vi "uc480_SubVI_Example_GetImageSize.vi"(8 "Error In":errorcluster, 11 ".NET (Reference)":refnum<k24>) -> (0 "Error Out":errorcluster, 1 "Height":i32, 2 "Width":i32, 3 ".NET (Reference)":refnum<k24>)   [LabVIEW 2011]
uses:
  C:/Program Files/Thorlabs/Scientific Imaging/DCx Camera Support/Develop/DotNet/uc480DotNet.dll
  Develop/DotNet/uc480DotNet.dll
panel:
  out "SubSampFacVert":i32
  out "Subsampled Width":i32
  out "Binned Width":i32
  out "Subsampled Height":i32
  out "SubSampFacHor":i32
  out "Factored Width":i32
  out "Factored Height":i32
  out "Binned Height":i32
  out "Scaler":dbl
  out "BinFacVert":i32
  out "BinFaHor":i32
  out "bAbsPosY":bool
  out "bAbsPosX":bool
  out "Max Width":i32
  out "Max Height":i32
  out "s32PosY":i32
  out "s32PosX":i32
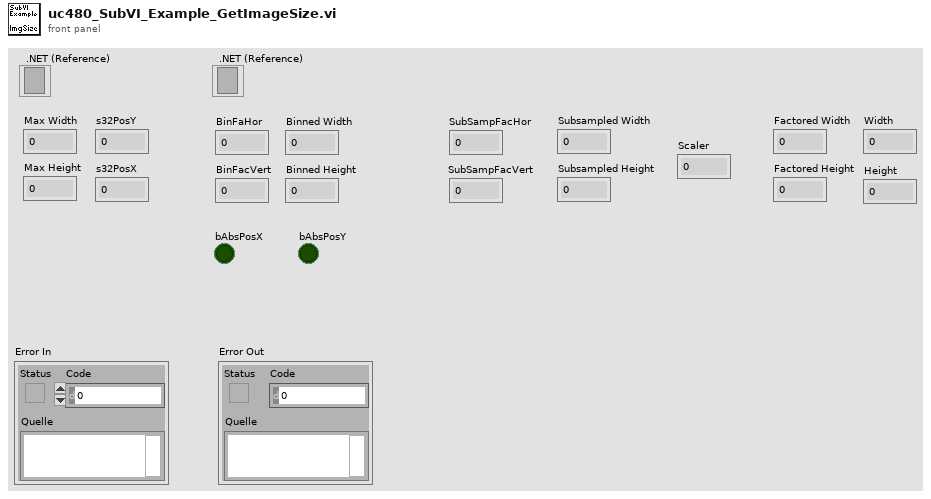
[diagram p1: front panel]
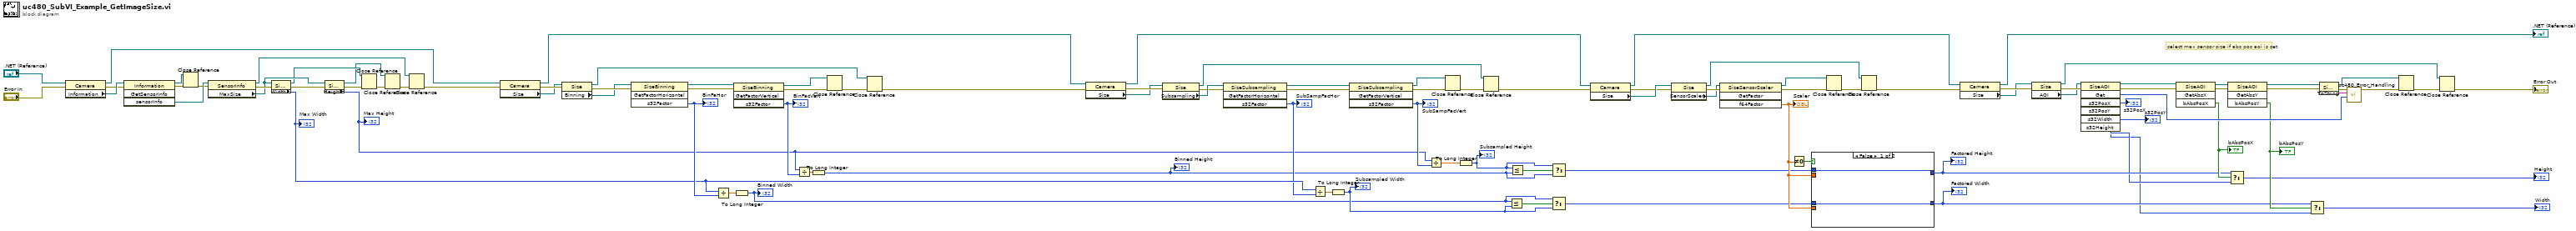
[diagram p0: block diagram]
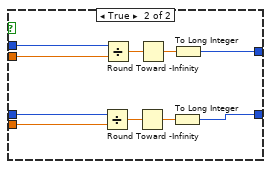
[diagram p2: hidden frame]
diagram:
  # "select max sensor size if abs pos aoi is set"
  n1 = property class="Camera"(reference=".NET (Reference)", error in="Error In") -> (reference out=w33:refnum<k24>, error out=w96:errorcluster, "Information"=w98:refnum<k24>)
  n2 = invoke class="Information" method="GetSensorInfo"(reference=w98, error in=w96) -> (reference out=w37:refnum<k24>, error out=w38:errorcluster, "sensorInfo"=w97:refnum<k24>)  [unwired: 2 in, 1 out]
  n3 = Close Reference(reference=w37, error in (no error)=w38) -> (error out=w39:errorcluster)
  n4 = property class="SensorInfo"(reference=w97, error in=w39) -> (reference out=w34:refnum<k24>, error out=w95:errorcluster, "MaxSize"=w44:refnum<k24>)
  n5 = property class="Size`1[[System.Int32, mscorlib,"(reference=w44, error in=w95) -> (reference out=w43:refnum<k24>, error out=w94:errorcluster, "Width"=w61:i32)
  "Max Width" <- w61
  n6 = property class="Size`1[[System.Int32, mscorlib,"(reference=w44, error in=w94) -> (reference out=w42:refnum<k24>, error out=w41:errorcluster, "Height"=w58:i32)
  "Max Height" <- w58
  n7 = Close Reference(reference=w43, error in (no error)=w41) -> (error out=w40:errorcluster)
  n8 = Close Reference(reference=w42, error in (no error)=w40) -> (error out=w36:errorcluster)
  n9 = Close Reference(reference=w34, error in (no error)=w36) -> (error out=w35:errorcluster)
  n10 = property on="Eigenschaftsknoten" class="Camera"(reference=w33, error in=w35) -> (reference out=w31:refnum<k24>, error out=w73:errorcluster, "Size"=w49:refnum<k24>)
  n11 = property class="Size"(reference=w49, error in=w73) -> (reference out=w27:refnum<k24>, error out=w82:errorcluster, "Binning"=w81:refnum<k24>)
  n12 = invoke class="SizeBinning" method="GetFactorHorizontal"(reference=w81, error in=w82) -> (reference out=w25:refnum<k24>, error out=w32:errorcluster, "s32Factor"=w62:i32)  [unwired: 2 in, 1 out]
  "BinFaHor" <- w62
  n13 = Divide(x=w61, y=w62) -> (x/y=w65:dbl)
  n14 = invoke class="SizeBinning" method="GetFactorVertical"(reference=w25, error in=w32) -> (reference out=w28:refnum<k24>, error out=w29:errorcluster, "s32Factor"=w63:i32)  [unwired: 2 in, 1 out]
  "BinFacVert" <- w63
  n15 = To Long Integer(number=w65) -> (32bit integer=w52:i32)
  "Binned Width" <- w52
  n16 = Divide(x=w58, y=w63) -> (x/y=w78:dbl)
  n17 = To Long Integer(number=w78) -> (32bit integer=w55:i32)
  "Binned Height" <- w55
  n18 = Close Reference(reference=w28, error in (no error)=w29) -> (error out=w24:errorcluster)
  n19 = Close Reference(reference=w27, error in (no error)=w24) -> (error out=w26:errorcluster)
  n20 = property on="Eigenschaftsknoten" class="Camera"(reference=w31, error in=w26) -> (reference out=w20:refnum<k24>, error out=w30:errorcluster, "Size"=w16:refnum<k24>)
  n21 = property class="Size"(reference=w16, error in=w30) -> (reference out=w15:refnum<k24>, error out=w69:errorcluster, "Subsampling"=w72:refnum<k24>)
  n22 = invoke class="SizeSubsampling" method="GetFactorHorizontal"(reference=w72, error in=w69) -> (reference out=w70:refnum<k24>, error out=w71:errorcluster, "s32Factor"=w59:i32)  [unwired: 2 in, 1 out]
  "SubSampFacHor" <- w59
  n23 = Divide(x=w61, y=w59) -> (x/y=w64:dbl)
  n24 = To Long Integer(number=w64) -> (32bit integer=w53:i32)
  "Subsampled Width" <- w53
  n25 = invoke class="SizeSubsampling" method="GetFactorVertical"(reference=w70, error in=w71) -> (reference out=w22:refnum<k24>, error out=w23:errorcluster, "s32Factor"=w60:i32)  [unwired: 2 in, 1 out]
  "SubSampFacVert" <- w60
  n26 = Divide(x=w58, y=w60) -> (x/y=w68:dbl)
  n27 = Close Reference(reference=w22, error in (no error)=w23) -> (error out=w18:errorcluster)
  n28 = To Long Integer(number=w68) -> (32bit integer=w56:i32)
  "Subsampled Height" <- w56
  n29 = Close Reference(reference=w15, error in (no error)=w18) -> (error out=w17:errorcluster)
  n30 = Less Or Equal?(x=w52, y=w53) -> (x <= y?=w54:bool)
  n31 = Less Or Equal?(x=w56, y=w55) -> (x <= y?=w57:bool)
  n32 = Select(t=w52, s=w54, f=w53) -> (s? t:f=w50:i32)
  n33 = Select(t=w56, s=w57, f=w55) -> (s? t:f=w51:i32)
  n34 = property on="Eigenschaftsknoten" class="Camera"(reference=w20, error in=w17) -> (reference out=w12:refnum<k24>, error out=w19:errorcluster, "Size"=w21:refnum<k24>)
  n35 = property class="Size"(reference=w21, error in=w19) -> (reference out=w7:refnum<k24>, error out=w80:errorcluster, "SensorScaler"=w79:refnum<k24>)
  n36 = invoke class="SizeSensorScaler" method="GetFactor"(reference=w79, error in=w80) -> (reference out=w9:refnum<k24>, error out=w10:errorcluster, "f64Factor"=w67:dbl)  [unwired: 2 in, 1 out]
  "Scaler" <- w67
  n37 = Not Equal To 0?(x=w67) -> (x != 0?=w66:bool)
  n38 = case shown="False" w66 {
    tunnel: w51 -> [w104 w108]
    tunnel: w50 -> [w103 w106]
    tunnel: w67 -> [_ w107]
    tunnel: w67 -> [_ w105]
    tunnel: [w104 w110] -> w76
    tunnel: [w103 w109] -> w75
    frame False {
    }
    frame True {
      n39 = Divide(x=w106, y=w105) -> (x/y=w111:dbl)
      n40 = Divide(x=w108, y=w107) -> (x/y=w114:dbl)
      n41 = Round Toward -Infinity(1:w111) -> (0:w112:dbl)
      n42 = Round Toward -Infinity(1:w114) -> (0:w113:dbl)
      n43 = To Long Integer(number=w112) -> (32bit integer=w109:i32)
      n44 = To Long Integer(number=w113) -> (32bit integer=w110:i32)
    }
  }
  "Factored Height" <- w76
  "Factored Width" <- w75
  n45 = Close Reference(reference=w9, error in (no error)=w10) -> (error out=w8:errorcluster)
  n46 = Close Reference(reference=w7, error in (no error)=w8) -> (error out=w6:errorcluster)
  n47 = property on="Eigenschaftsknoten" class="Camera"(reference=w12, error in=w6) -> (reference out=→".NET (Reference)":refnum<k24>, error out=w14:errorcluster, "Size"=w13:refnum<k24>)
  n48 = property class="Size"(reference=w13, error in=w14) -> (reference out=w2:refnum<k24>, error out=w84:errorcluster, "AOI"=w83:refnum<k24>)
  n49 = invoke class="SizeAOI" method="Get"(reference=w83, error in=w84) -> (reference out=w93:refnum<k24>, error out=w90:errorcluster, "Get"=w87:i32, "s32PosX"=→"s32PosX":i32, "s32PosY"=→"s32PosY":i32, "s32Width"=w45:i32, "s32Height"=w46:i32)  [unwired: 5 in]
  n50 = invoke class="SizeAOI" method="GetAbsX"(reference=w93, error in=w90) -> (reference out=w92:refnum<k24>, error out=w91:errorcluster, "bAbsPosX"=w86:bool)  [unwired: 2 in, 1 out]
  "bAbsPosX" <- w86
  n51 = invoke class="SizeAOI" method="GetAbsY"(reference=w92, error in=w91) -> (reference out=w89:refnum<k24>, error out=w88:errorcluster, "bAbsPosY"=w85:bool)  [unwired: 2 in, 1 out]
  "bAbsPosY" <- w85
  n52 = Select(t=w76, s=w86, f=w46) -> (s? t:f=→"Height":i32)
  n53 = Select(t=w75, s=w85, f=w45) -> (s? t:f=→"Width":i32)
  n54 = invoke class="SizeAOI" method="ToString"(reference=w89, error in=w88) -> (reference out=w4:refnum<k24>, error out=w101:errorcluster, "ToString"=w102:string)  [unwired: 1 in]
  n55 = call "uc480_Error_Handling.vi"("Error Code"=w87, "Error String"=w102, "Error In"=w101) -> ("Error Out"=w5:errorcluster)  [unwired: 8 in]
  n56 = Close Reference(reference=w4, error in (no error)=w5) -> (error out=w3:errorcluster)
  n57 = Close Reference(reference=w2, error in (no error)=w3) -> (error out=→"Error Out":errorcluster)
